vi "Is Pause Elapsed.vi"(8 "error in (no error)":errorcluster, 11 "Spectrum Recorder too in":refnum<class "Spectrum Recorder too.lvclass">) -> (0 "error out":errorcluster, 1 "Input finish":bool, 2 "Start new scan":bool, 3 "Spectrum Recorder too out":refnum<class "Spectrum Recorder too.lvclass">, 4 "pause":bool, 5 "Reset":bool, 6 "Restart time":timestamp, 7 "Input finish time":timestamp)   [LabVIEW 2020, in "Spectrum Recorder too.lvclass"]
uses:
  Spectrum Recorder too.lvclass
  Spectrum Recorder too.lvclass/Spectrum Recorder too.ctl
  Read Spectrum Recorder Configuration.vi
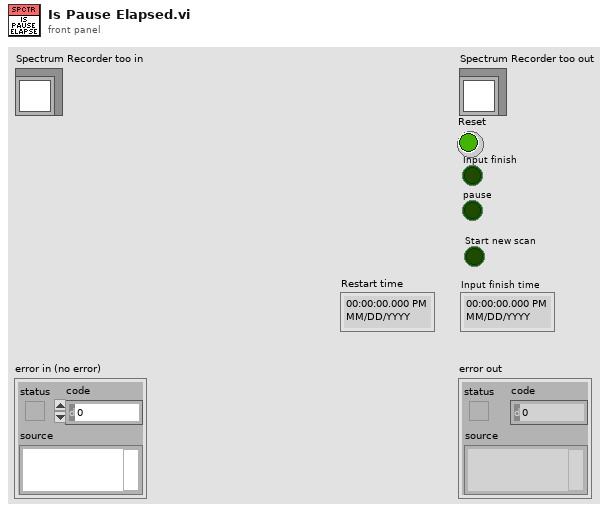
[diagram p1: front panel]
types:
  T1 = typedef "Spectrum Configuration.ctl" = cluster{"Start frequency":dbl, "End frequency":dbl, "Coarse step":dbl, "Step duration":dbl, "Red Pitaya address":string, "Open plot \non start":bool, "Regions width":dbl, "Fine step":dbl, "Pause between scans":dbl, "Clear rgs on start":bool, "Output amplitude":dbl, "Append measurements":string[]}
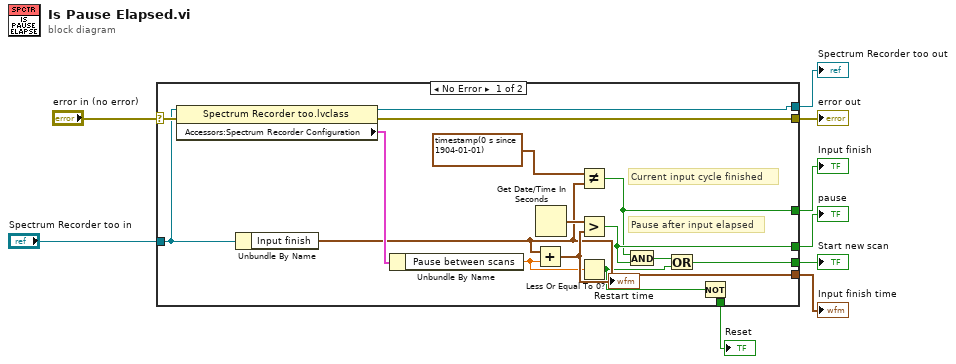
[diagram p0: block diagram]
diagram:
  n1 = case shown="No Error" "error in (no error)" {
    selector: "error in (no error)" -> [w19 w27]
    tunnel: [w16 w27] -> w8
    tunnel: [w18 w26] -> w6
    tunnel: "Spectrum Recorder too in" -> [w17 w26]
    tunnel: [w15 _] -> w5
    tunnel: [w14 _] -> w4
    tunnel: [w13 _] -> w3
    tunnel: [w12 _] -> w2
    tunnel: [w10 _] -> w1
    frame No Error {
      # "Pause after input elapsed"
      # "Current input cycle finished"
      n2 = property class="Spectrum Recorder too.lvclass"(reference=w17, error in=w19) -> (reference out=w18:refnum<class "Spectrum Recorder too.lvclass">, error out=w16:errorcluster, "Accessors:Spectrum Recorder Configuration"=w21:T1)
      n3 = Unbundle By Name(w17) -> ("Input finish"=w12:timestamp)
      n4 = Unbundle By Name(w21) -> ("Pause between scans"=w22:dbl)
      n5 = Add(x=w12, y=w22) -> (x+y=w24:timestamp)
      "Restart time" <- w24
      n6 = Get Date/Time In Seconds() -> (seconds since 1Jan1904=w23:timestamp)
      n7 = Not Equal?(x=timestamp(0 s since 1904-01-01), y=w12) -> (x != y?=w13:bool)
      n8 = Greater?(x=w23, y=w24) -> (0:w14:bool)
      n9 = Less Or Equal To 0?(x=w22) -> (x <= 0?=w11:bool)
      n10 = And(x=w13, y=w14) -> (x .and. y?=w25:bool)
      n11 = Or(x=w25, y=w11) -> (x .or. y?=w15:bool)
      n12 = Not(x=w11) -> (.not. x?=w10:bool)
    }
    frame Error {
    }
  }
  "error out" <- w8
  "Spectrum Recorder too out" <- w6
  "Start new scan" <- w5
  "pause" <- w4
  "Input finish" <- w3
  "Input finish time" <- w2
  "Reset" <- w1
